vi "process.vi"(8 "error in":errorcluster, 9 "result allocation":T1, 10 "parameters":T1, 11 "module in":refnum<class "Benchmark PID runtime.lvclass">) -> (0 "error out":errorcluster, 1 "results":T1, 2 "parameter allocation":T1, 3 "module out":refnum<class "Benchmark PID runtime.lvclass">)   [LabVIEW 2018, in "Benchmark PID runtime.lvclass"]
doc: "Provides an interface for information processing by a module at runtime. While this interface performs no operations, a child should provide an override which may process data in any manner necessary."
uses:
  Benchmark PID runtime.lvclass
  <vilib>/NI/Tag Bus/table/data table.ctl
  Benchmark PID runtime.lvclass/Benchmark PID runtime.ctl
  <vilib>/NI/Tag Bus/table/data polymorphs/read one/read Double.vi
  <vilib>/NI/Tag Bus/table/data polymorphs/write one/write Double.vi
  <vilib>/addons/control/pid/pid.llb/PID (DBL).vi
  <vilib>/addons/control/pid/NI_PID_pid.lvlib
  <vilib>/NI/Tag Bus/table/data table.lvlib
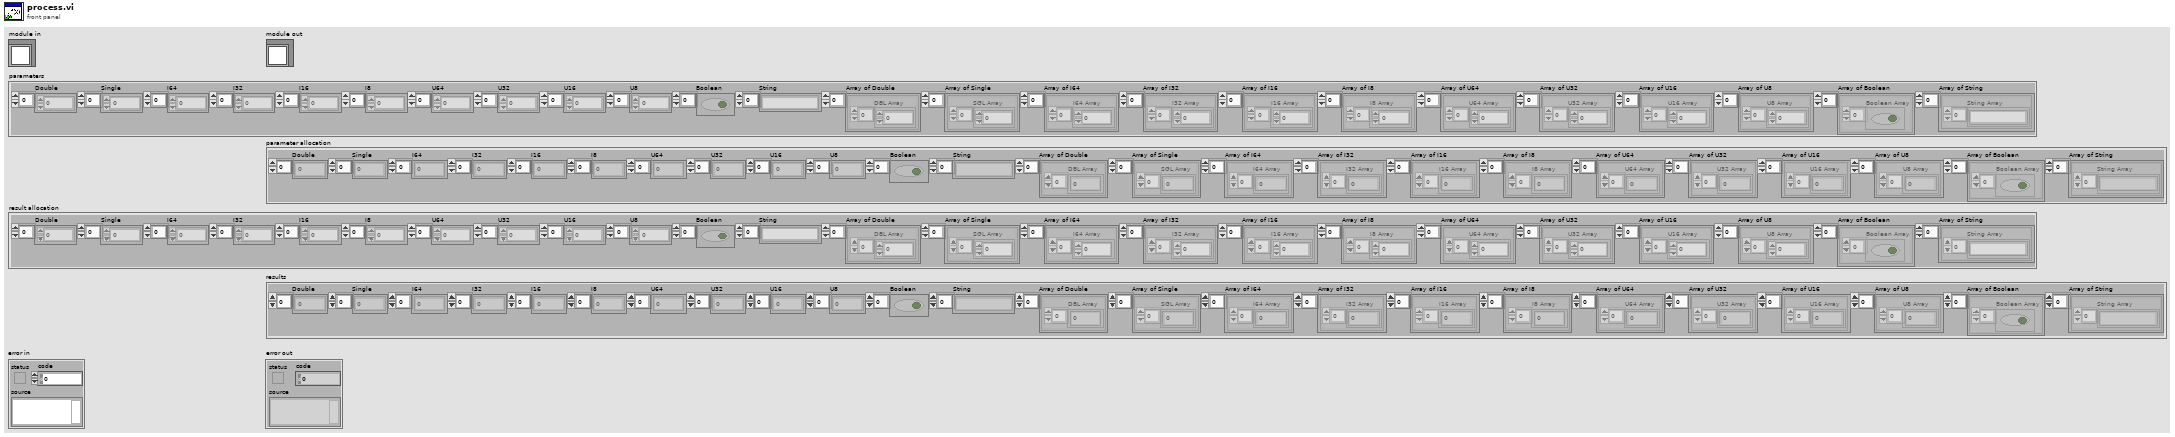
[diagram p1: front panel]
types:
  T1 = typedef "tag bus.lvlib/data table.lvlib/data table.ctl" = cluster{"Double":dbl[], "Single":sgl[], "I64":i64[], "I32":i32[], "I16":i16[], "I8":i8[], "U64":u64[], "U32":u32[], "U16":u16[], "U8":u8[], "Boolean":bool[], "String":string[], "Array of Double":cluster{"DBL Array":dbl[]}[], "Array of Single":cluster{"SGL Array":sgl[]}[], "Array of I64":cluster{"I64 Array":i64[]}[], "Array of I32":cluster{"I32 Array":i32[]}[], "Array of I16":cluster{"I16 Array":i16[]}[], "Array of I8":cluster{"I8 Array":i8[]}[], "Array of U64":cluster{"U64 Array":u64[]}[], "Array of U32":cluster{"U32 Array":u32[]}[], "Array of U16":cluster{"U16 Array":u16[]}[], "Array of U8":cluster{"U8 Array":u8[]}[], "Array of Boolean":cluster{"Boolean Array":bool[]}[], "Array of String":cluster{"String Array":string[]}[]}
  T2 = typedef "Mappings.ctl" = cluster{"Setpoint Index":i32, "Variable Index":i32, "Output Index":i32}
  T3 = cluster{"proportional gain (Kc)":dbl, "integral time (Ti, min)":dbl, "derivative time (Td, min)":dbl}
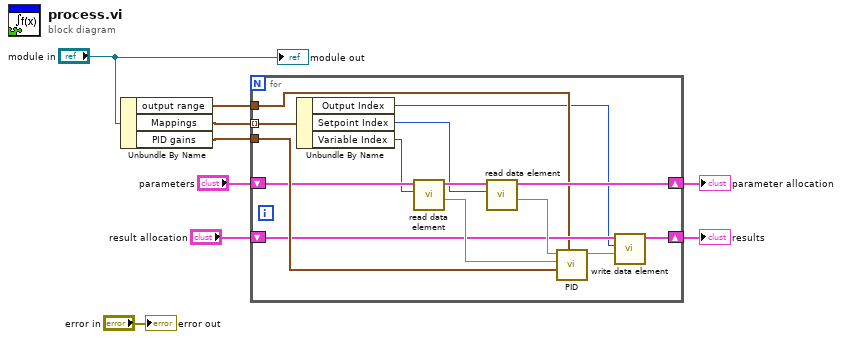
[diagram p0: block diagram]
diagram:
  n1 = Unbundle By Name("module in") -> ("output range"=w1:cluster{"output high":dbl, "output low":dbl}, "Mappings"=w2:T2[], "PID gains"=w9:T3)
  n2 = for {
    tunnel: w9 -> [w23]
    tunnel: w2 -> [w22] mode=indexing
    shift-right: [w18] -> w7
    shift-left: "result allocation" -> [w19]
    shift-right: [w15] -> w6
    shift-left: "parameters" -> [w14]
    tunnel: w1 -> [w13]
    n3 = Unbundle By Name(w22) -> ("Output Index"=w10:i32, "Setpoint Index"=w11:i32, "Variable Index"=w12:i32)
    n4 = call-poly <vilib>:"read data element.vi"("index"=w12, "data table in"=w14) -> ("value"=w20:dbl, "data table out"=w16:T1)  [unwired: 8 in]
    n5 = call-poly <vilib>:"read data element.vi"("index"=w11, "data table in"=w16) -> ("value"=w21:dbl, "data table out"=w15:T1)  [unwired: 8 in]
    n6 = call-poly <vilib>:"PID.vi"("output range"=w13, "PID gains"=w23, "process variable"=w20, "setpoint"=w21) -> ("output"=w17:dbl)  [unwired: 6 in, 1 out]
    n7 = call-poly <vilib>:"write data element.vi"("value"=w17, "index"=w10, "data table in"=w19) -> ("data table out"=w18:T1)  [unwired: 8 in]
  }
  "results" <- w7
  "parameter allocation" <- w6
  "error out" <- "error in"
  "module out" <- "module in"
